vi "DAQ wait.vi"(7 "DAQ state cluster in":T1={"DAQ state"=enum."Global comm", "device"="", "start (ms)"=0, "error"={"status"=FALSE, "code"=0, "source"=""}, "T cont"={"exec"={"T mode"=enum."Listening to exec", "man power"=0.0, "log"=FALSE}, "T status"={"Temp"=0.0, "Power"=0.0}, "utility"={"meas index"=0, "wait (ms)"=0, "H Vmax"=8.5, "power out"=5.0, "heat volt out"=0.0, "heat volt in"=0.0, "therm volt"=0.0, "t T P hist"=[]}}} {"T cont"."utility"."therm volt" format="%_6g"; "T cont"."utility"."heat volt in" format="%_6g"; "T cont"."utility"."heat volt out" format="%_6g"; "T cont"."utility"."power out" format="%_6g"; "T cont"."utility"."H Vmax" format="%_6g"; "T cont"."exec"."man power" format="%_6g"; "T cont"."T status"."Power" format="%_6g"; "T cont"."T status"."Temp" format="%_6g"}) -> (8 "DAQ state cluster out":T1={"DAQ state"=enum."Global comm", "device"="", "start (ms)"=0, "error"={"status"=FALSE, "code"=0, "source"=""}, "T cont"={"exec"={"T mode"=enum."Listening to exec", "man power"=0.0, "log"=FALSE}, "T status"={"Temp"=0.0, "Power"=0.0}, "utility"={"meas index"=0, "wait (ms)"=0, "H Vmax"=8.5, "power out"=5.0, "heat volt out"=0.0, "heat volt in"=0.0, "therm volt"=0.0, "t T P hist"=[]}}} {"T cont"."utility"."therm volt" format="%_6g"; "T cont"."utility"."heat volt in" format="%_6g"; "T cont"."utility"."heat volt out" format="%_6g"; "T cont"."utility"."power out" format="%_6g"; "T cont"."utility"."H Vmax" format="%_6g"; "T cont"."exec"."man power" format="%_6g"; "T cont"."T status"."Power" format="%_6g"; "T cont"."T status"."Temp" format="%_6g"})   [LabVIEW 2019]
doc: "This subVI is one of the states of the DAQ state machine in the bug experiment.\n\nThis state waits the time set in the state cluster, it returns to global comm.\n\nPaul K Dixon\nP3600\nCSUSB Physics"
uses:
  typedefs/DAQ T state cluster.ctl
  typedefs/DAQ T state enum.ctl
  typedefs/temp cont cluster.ctl
  typedefs/temp exec cluster.ctl
  typedefs/temp mode enum.ctl
  typedefs/temp indicator.ctl
  typedefs/temp cont utility.ctl
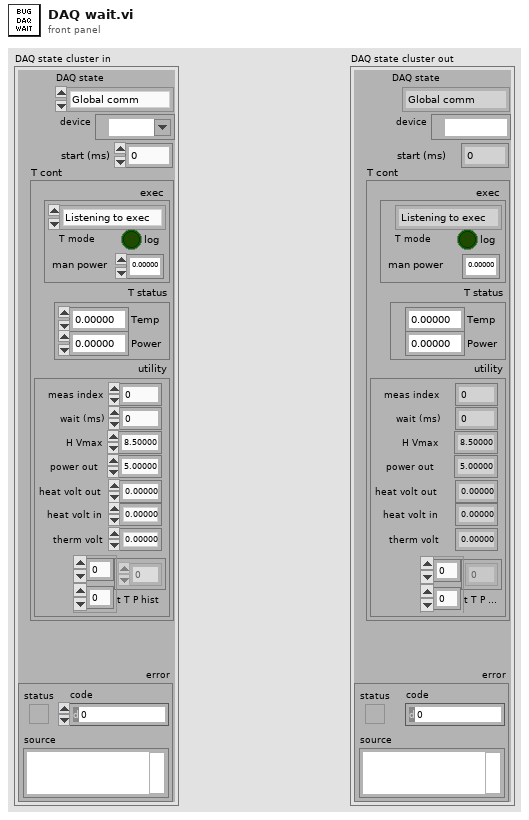
[diagram p1: front panel]
types:
  T1 = typedef "DAQ T state cluster.ctl" = cluster{"DAQ state":T2, "device":tag, "start (ms)":i32, "error":errorcluster, "T cont":T3}
  T2 = typedef "DAQ T state enum.ctl" = enum16{"Global comm", "Meas T & P", "Man Power set", "Output Power", "Wait", "Exit"}
  T3 = typedef "temp cont cluster.ctl" = cluster{"exec":T4, "T status":T6, "utility":T7}
  T4 = typedef "temp exec cluster.ctl" = cluster{"T mode":T5, "man power":dbl, "log":bool}
  T5 = typedef "temp mode enum.ctl" = enum16{"Setting up", "Listening to exec", "Exit"}
  T6 = typedef "temp indicator.ctl" = cluster{"Temp":dbl, "Power":dbl}
  T7 = typedef "temp cont utility.ctl" = cluster{"meas index":i32, "wait (ms)":i32, "H Vmax":dbl, "power out":dbl, "heat volt out":dbl, "heat volt in":dbl, "therm volt":dbl, "t T P hist":dbl[][]}
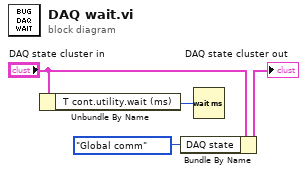
[diagram p0: block diagram]
diagram:
  n1 = Unbundle By Name("DAQ state cluster in") -> ("T cont.utility.wait (ms)"=w1:i32)
  n2 = Bundle By Name(cluster="DAQ state cluster in", "DAQ state"=DAQ_T_state_enum."Global comm") -> (→"DAQ state cluster out":T1)
  n3 = Wait (ms)(milliseconds to wait=w1) -> ()  [unwired: 1 out]
